vi "prep bdd init.vi"(10 "taille de la dimension":i32, 11 "3P4S?":bool) -> (3 "Tableau":string[](array[string]))   [LabVIEW 2020]
uses:
  CtrldeTest/selectdata.ctl
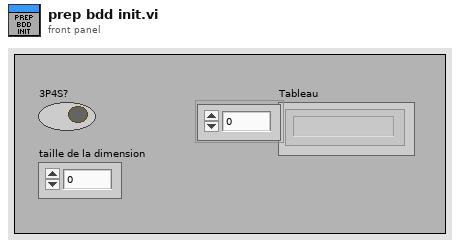
[diagram p1: front panel]
types:
  T1 = typedef "selectdata.ctl" = u16
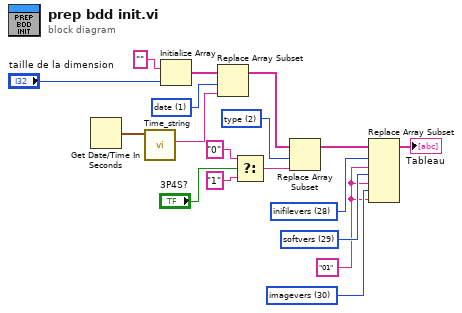
[diagram p0: block diagram]
diagram:
  w15 = T1 30 items=["id", "date", "type", "sn", "ocv", "acir", "insuP", "insuN", "TC01", "TC02", "TC11", "TC12", "TC21", "TC22", "VC01", "VC02", "VC03", "VC04", "VC11", "VC12", "VC13", "VC14", "VC21", "VC22", "VC23", "VC24", "DCIRN", "DCIRP", "inifilevers", "softvers", "imagevers", "pass", "operateur", "tpstest"] ("Menu déroulant")
  w14 = T1 29 items=["id", "date", "type", "sn", "ocv", "acir", "insuP", "insuN", "TC01", "TC02", "TC11", "TC12", "TC21", "TC22", "VC01", "VC02", "VC03", "VC04", "VC11", "VC12", "VC13", "VC14", "VC21", "VC22", "VC23", "VC24", "DCIRN", "DCIRP", "inifilevers", "softvers", "imagevers", "pass", "operateur", "tpstest"] ("Menu déroulant")
  w13 = "01" ("nouvel élément/sous-tableau")
  w8 = T1 28 items=["id", "date", "type", "sn", "ocv", "acir", "insuP", "insuN", "TC01", "TC02", "TC11", "TC12", "TC21", "TC22", "VC01", "VC02", "VC03", "VC04", "VC11", "VC12", "VC13", "VC14", "VC21", "VC22", "VC23", "VC24", "DCIRN", "DCIRP", "inifilevers", "softvers", "imagevers", "pass", "operateur", "tpstest"] ("Menu déroulant")
  w11 = T1 1 items=["id", "date", "type", "sn", "ocv", "acir", "insuP", "insuN", "TC01", "TC02", "TC11", "TC12", "TC21", "TC22", "VC01", "VC02", "VC03", "VC04", "VC11", "VC12", "VC13", "VC14", "VC21", "VC22", "VC23", "VC24", "DCIRN", "DCIRP", "inifilevers", "softvers", "imagevers", "pass", "operateur", "tpstest"] ("Menu déroulant")
  w3 = T1 2 items=["id", "date", "type", "sn", "ocv", "acir", "insuP", "insuN", "TC01", "TC02", "TC11", "TC12", "TC21", "TC22", "VC01", "VC02", "VC03", "VC04", "VC11", "VC12", "VC13", "VC14", "VC21", "VC22", "VC23", "VC24", "DCIRN", "DCIRP", "inifilevers", "softvers", "imagevers", "pass", "operateur", "tpstest"] ("Menu déroulant")
  n1 = Get Date/Time In Seconds() -> (seconds since 1Jan1904=w18:timestamp)
  n2 = call <userlib>:"Time_string.vi"("h in"=w18) -> ("heure sql"=w16:string)  [unwired: 9 in, 1 out]
  n3 = Initialize Array("", "taille de la dimension") -> (w10:string[])
  n4 = Replace Array Subset(array=w10, new element=w16, index=w11) -> (w12:string[])
  n5 = Select(t="0", s="3P4S?", f="1" ("cas faux")) -> (s? t:f=w4:string)
  n6 = Replace Array Subset(array=w12, new element=w4, index=w3) -> (w6:string[])
  n7 = Replace Array Subset(array=w6, new element #1=w13, index #1=w8, new element #2=w13, index #2=w14, new element #3=w13, index #3=w15) -> (→"Tableau":string[])
